vi "Highest Pixel Abscissa Determination.vi"(8 "error in":errorcluster, 9 "Column Number from Edge Detection VI":i32, 10 "Pin Width from Pixel Intensity Determination VI":i32, 11 "Image":T1) -> (0 "error out":errorcluster, 3 "Pixel Value - Maximum Gradient occurs":dbl)   [LabVIEW 2016]
uses:
  <vilib>/vision/Image Controls.llb/IMAQ Image.ctl
panel:
  out "Pixel Value - Left Limit":i32
  out "Pixel Value - Right Limit":i32
  out "Pixel Value - Limting Point":i32
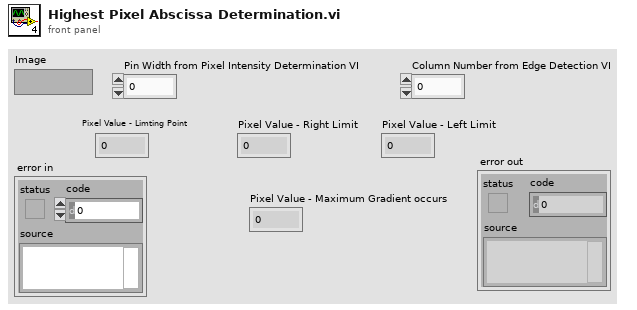
[diagram p1: front panel]
types:
  T1 = typedef "IMAQ Image.ctl" = refnum<image>
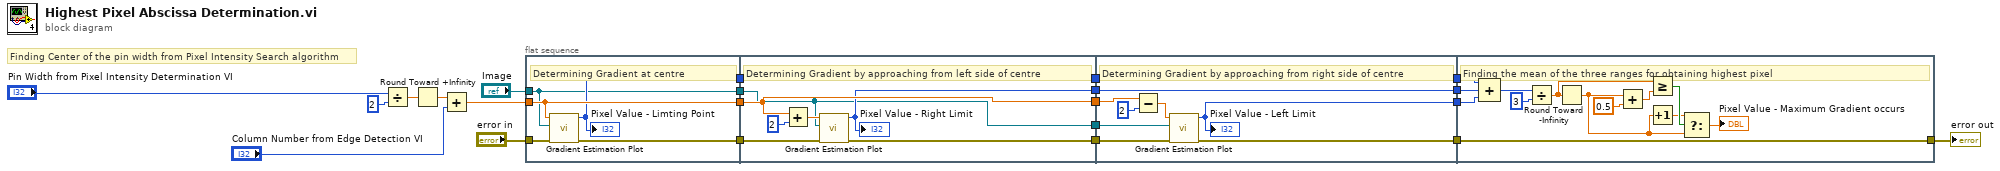
[diagram p0: block diagram]
diagram:
  # "Finding Center of the pin width from Pixel Intensity Search algorithm"
  n1 = Divide(x="Pin Width from Pixel Intensity Determination VI", y=2) -> (x/y=w10:dbl)
  n2 = Round Toward +Infinity(x=w10) -> (ceil(x): smallest int >= x=w8:dbl)
  n3 = Add(x=w8, y="Column Number from Edge Detection VI") -> (x+y=w7:dbl)
  n4 = flat-sequence {
    tunnel: w7 -> [w27]
    tunnel: [w27] -> w22
    tunnel: [w26] -> w21
    tunnel: [w25] -> w6
    tunnel: "error in" -> [w24]
    tunnel: "Image" -> [w23]
    tunnel: [w23] -> w2
    tunnel: w22 -> [w35]
    tunnel: [w35] -> w20
    tunnel: [w33] -> w19
    tunnel: w21 -> [w33]
    tunnel: [w30] -> w18
    tunnel: [w29] -> w17
    tunnel: w6 -> [w31]
    tunnel: w2 -> [w28]
    tunnel: [w28] -> w1
    tunnel: w20 -> [w44]
    tunnel: [w42] -> w16
    tunnel: w19 -> [w42]
    tunnel: w18 -> [w39]
    tunnel: [w38] -> w15
    tunnel: w17 -> [w41]
    tunnel: [w41] -> w14
    tunnel: [w37] -> w13
    tunnel: w1 -> [w36]
    tunnel: w16 -> [w57]
    tunnel: w15 -> [w47]
    tunnel: [w47] -> w5
    tunnel: w14 -> [w46]
    tunnel: w13 -> [w45]
    frame #0 {
      # "Determining Gradient at centre"
      n5 = call "Gradient Estimation Plot.vi"("error in"=w24, "Image"=w23, "Pixel Column Number from edge detection"=w27) -> ("error out"=w25:errorcluster, "Value of Pixel at which maximum gradient occurs"=w26:i32)  [unwired: 7 in]
      "Pixel Value - Limting Point" <- w26
    }
    frame #1 {
      # "Determining Gradient by approaching from left side of centre"
      n6 = Add(x=w35, y=2) -> (x+y=w32:dbl)
      n7 = call "Gradient Estimation Plot.vi"("error in"=w31, "Image"=w28, "Pixel Column Number from edge detection"=w32) -> ("error out"=w30:errorcluster, "Value of Pixel at which maximum gradient occurs"=w29:i32)  [unwired: 7 in]
      "Pixel Value - Right Limit" <- w29
    }
    frame #2 {
      # "Determining Gradient by approaching from right side of centre"
      n8 = Subtract(x=w44, y=2) -> (x-y=w40:dbl)
      n9 = call "Gradient Estimation Plot.vi"("error in"=w39, "Image"=w36, "Pixel Column Number from edge detection"=w40) -> ("error out"=w38:errorcluster, "Value of Pixel at which maximum gradient occurs"=w37:i32)  [unwired: 7 in]
      "Pixel Value - Left Limit" <- w37
    }
    frame #3 {
      # "Finding the mean of the three ranges for obtaining highest pixel"
      n10 = Compound Arithmetic op=ADD(w57, w46, w45) -> (w56:i32)
      n11 = Divide(x=w56, y=3) -> (x/y=w54:dbl)
      n12 = Round Toward -Infinity(1:w54) -> (0:w50:dbl)
      n13 = Add(x=w50, y=0.5) -> (x+y=w49:dbl)
      n14 = Greater Or Equal?(x=w54, y=w49) -> (x >= y?=w53:bool)
      n15 = Increment(x=w50) -> (x+1=w52:dbl)
      n16 = Select(t=w52, s=w53, f=w50) -> (s? t:f=→"Pixel Value - Maximum Gradient occurs":dbl)
    }
  }
  "error out" <- w5
